vi "Get Synced Projects.vi"(8 "Error In":errorcluster, 11 "Source Root":path=path "C:/github/labviewhacker") -> (0 "Error Out":errorcluster, 2 "Config File Paths":path[](array[path]), 3 "Synced Projects":string[](array[string]))   [LabVIEW 2011, in "LVH-Build-Tools.lvlib"]
uses:
  <vilib>/LabVIEW Hacker/Build Tools/LVH-Build-Tools.lvlib
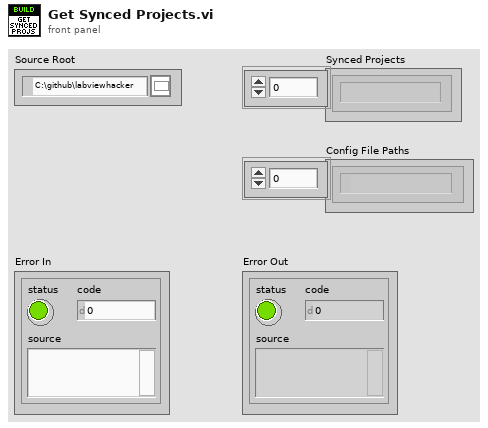
[diagram p1: front panel]
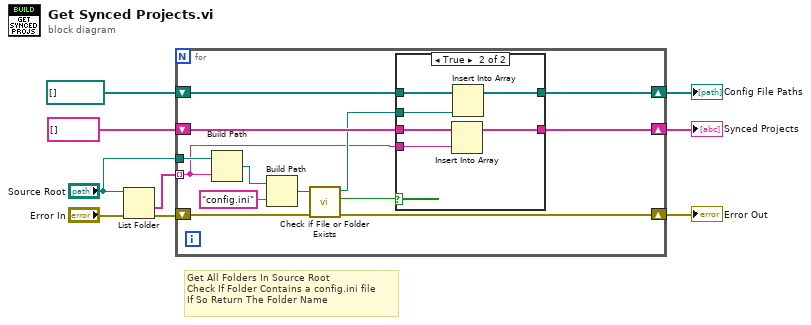
[diagram p0: block diagram]
diagram:
  # "Get All Folders In Source Root\nCheck If Folder Contains a config.ini file\nIf So Return The Folder Name"
  n1 = List Folder(path="Source Root", error in="Error In") -> (folder names=w8:string[], error out=w7:errorcluster)  [unwired: 2 in, 2 out]
  n2 = for {
    tunnel: "Source Root" -> [w22]
    tunnel: w8 -> [w10] mode=indexing
    shift-right: [w17] -> w5
    shift-left: w7 -> [w18]
    shift-right: [w14] -> w3
    shift-left: string[] [] -> [w16]
    shift-right: [w12] -> w1
    shift-left: path[] [] -> [w13]
    n3 = Build Path(base path=w22, name or relative path=w10) -> (appended path=w21:path)
    n4 = Build Path(base path=w21, name or relative path="config.ini") -> (appended path=w19:path)
    n5 = call <vilib>:"Check if File or Folder Exists.vi"("error in (no error)"=w18, "path"=w19) -> ("error out"=w17:errorcluster, "file or folder exists?"=w15:bool, "dup path"=w11:path)  [unwired: 7 in]
    n6 = case shown="True" w15 {
      tunnel: w16 -> [w24 w30]
      tunnel: [w24 w28] -> w14
      tunnel: w10 -> [_ w29]
      tunnel: w13 -> [w23 w27]
      tunnel: [w23 w26] -> w12
      tunnel: w11 -> [_ w25]
      frame False {
      }
      frame True {
        n7 = Insert Into Array(array=w30, new element=w29) -> (w28:string[])  [unwired: 1 in]
        n8 = Insert Into Array(array=w27, new element=w25) -> (w26:path[])  [unwired: 1 in]
      }
    }
  }
  "Error Out" <- w5
  "Synced Projects" <- w3
  "Config File Paths" <- w1
